vi "GenerateRandomNumberArray.vi"(1 "Size":dbl) -> (0 "Array":dbl[](array[numeric]))   [LabVIEW 2025, in "Utilities.lvlib" / "Random.lvlib"]
uses:
  Random.lvlib
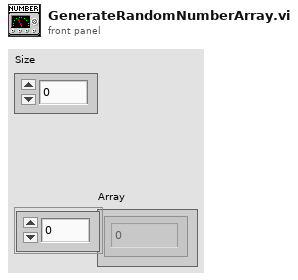
[diagram p1: front panel]
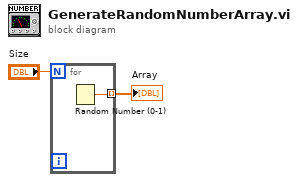
[diagram p0: block diagram]
diagram:
  n1 = for {
    N: "Size" -> [_]
    tunnel: [w3] -> w2 mode=indexing
    n2 = Random Number (0-1)() -> (number: 0 to 1=w3:dbl)
  }
  "Array" <- w2
